vi "AudioIN.vi"   [LabVIEW 2016]
uses:
  <vilib>/rvi/Emulation/niFpgaSctlEmulationGetInTimedLoop.vi
  <vilib>/rvi/eio/common/nirviEmuTemplateMethod_errors.vi
  Global 1.vi
  <vilib>/rvi/Emulation/niFpgaProcessEmulError.vi
  <vilib>/eio/EIONode/EIONode.xnode
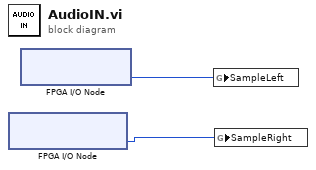
[diagram p0: block diagram]
diagram:
  n1 = xnode "FPGA I/O Node"() -> ("AudioIn/Right"=w1:i16)  [unwired: 1 in, 1 out]
  n2 = xnode "FPGA I/O Node"() -> ("AudioIn/Left"=w2:i16)  [unwired: 1 in, 1 out]
  n3 = global write "Global 1.vi" "SampleLeft"(w2) -> ()
  n4 = global write "Global 1.vi" "SampleRight"(w1) -> ()
